vi "Set_Time.vi"(1 "Time":dbl, 2 "Index":i32, 3 "Input Sequence":cluster{string, string[], dbl[], dbl}[](array[cluster])) -> (0 "Output Sequence":cluster{string, string[], dbl[], dbl}[](array[cluster]))   [LabVIEW 2011]
doc: "This VI sets the time value (in seconds) of an event in the sequence given by the \"Index\" parameter. The time value is analagous to the duration of a given event."
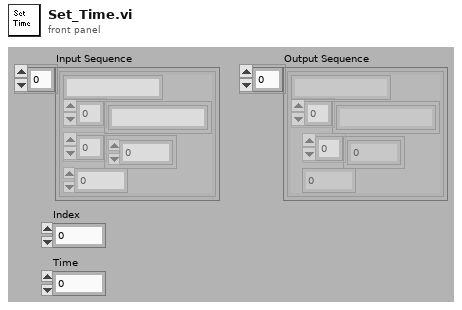
[diagram p1: front panel]
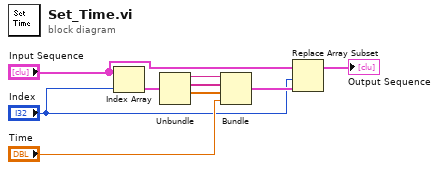
[diagram p0: block diagram]
diagram:
  n1 = Index Array(array="Input Sequence", index="Index") -> (element=w9:cluster{string, string[], dbl[], dbl})
  n2 = Unbundle(w9) -> (w8:string, w7:string[], w6:dbl[])  [unwired: 1 out]
  n3 = Bundle(w8, w7, w6, "Time"="Time") -> (w4:cluster{string, string[], dbl[], "Time":dbl})  [unwired: 1 out]
  n4 = Replace Array Subset(array="Input Sequence", new element=w4, index="Index") -> (→"Output Sequence":cluster{string, string[], dbl[], dbl}[])
